vi "Yokogawa Class Chooser.vi"(8 "Incoming Otpion":string, 9 "Incoming ID":string, 10 "VISA resource name":refnum<visa-resource-name>) -> (3 "Class out":refnum<class "Universal Power Meter.lvclass">)   [LabVIEW 2014, in "Universal Power Meter.lvlib" / "Universal Power Meter.lvclass"]
uses:
  Universal Power Meter.lvclass
panel:
  out "Model 2":string
  in  "error in (no error)":errorcluster
  out "error out":errorcluster
  out "Model":string
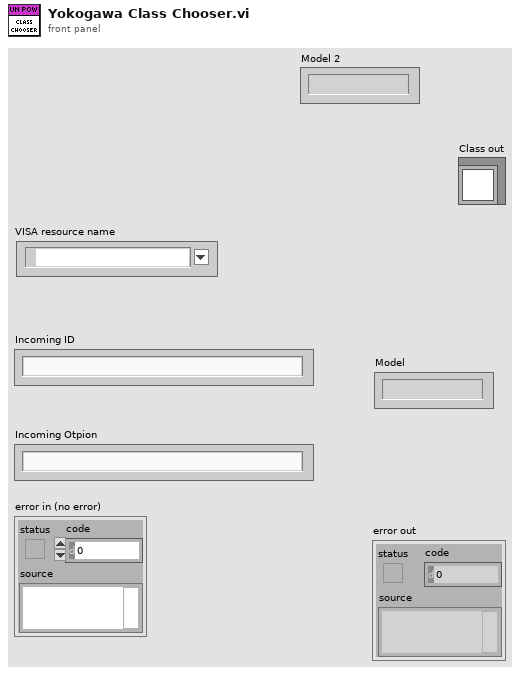
[diagram p1: front panel]
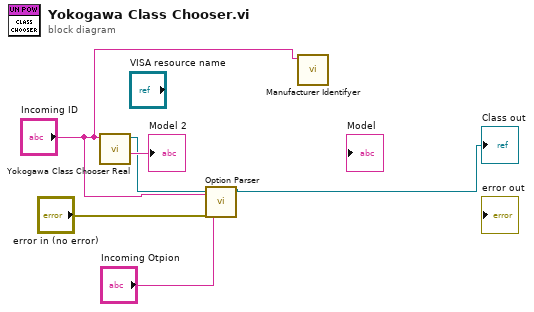
[diagram p0: block diagram]
diagram:
  n1 = call "Yokogawa Class Chooser Real.vi"("Incoming ID in"="Incoming ID") -> ("Model"=→"Model 2":string, "Universal Power Meter out"=w4:refnum<class "Universal Power Meter.lvclass">)  [unwired: 8 in, 1 out]
  n2 = call-dynamic "Option Parser.vi"("Universal Power Meter in"=w4, "ID"="Incoming ID", "error in (no error)"="error in (no error)", "Option"="Incoming Otpion") -> ("Universal Power Meter out"=→"Class out":refnum<class "Universal Power Meter.lvclass">)  [unwired: 14 in, 1 out]
  n3 = call "Manufacturer Identifyer.vi"("Visa In"="Incoming ID") -> ()  [unwired: 9 in, 2 out]
